vi "环动报警队列存储.vi"   [LabVIEW 2016, in "环境动力监测库.lvlib"]
types:
  T1 = cluster{"时间标识":timestamp, "设备":string, "日志信息":string}
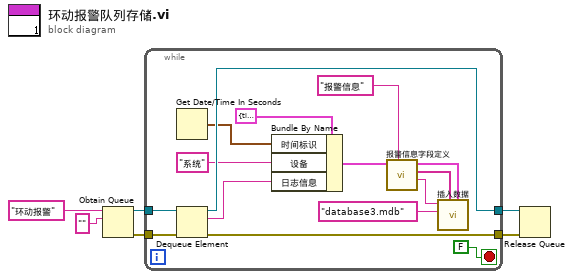
[diagram p0: block diagram]
diagram:
  n1 = Obtain Queue(name (unnamed)="环动报警" ("名称（未命名）"), element data type="" ("报警内容")) -> (queue out=w6:refnum<queue>, error out=w5:errorcluster)  [unwired: 3 in, 1 out]
  n2 = while {
    tunnel: w6 -> [w21]
    tunnel: w5 -> [w20]
    tunnel: [w18] -> w3
    tunnel: [w17] -> w2
    stop <- FALSE stop-if-true
    n3 = Get Date/Time In Seconds() -> (seconds since 1Jan1904=w9:timestamp)
    n4 = Dequeue Element(queue=w21, error in (no error)=w20) -> (queue out=w18:refnum<queue>, element=w7:string, error out=w17:errorcluster)  [unwired: 1 in, 1 out]
    n5 = Bundle By Name(cluster=T1 {"时间标识"=timestamp(0 s since 1904-01-01), "设备"="", "日志信息"=""} ("data in"), "时间标识"=w9, "设备"="系统", "日志信息"=w7) -> (w10:T1)
    n6 = call "报警信息字段定义.vi"("table输入"="报警信息", "data in"=w10) -> ("table输出"=w14:string, "columns"=w15:string[], "data out"=w16:T1)  [unwired: 7 in]
    n7 = call "插入数据.vi"("data"=w16, "columns"=w15, "database"="database3.mdb", "table"=w14) -> ()  [unwired: 7 in, 1 out]
  }
  n8 = Release Queue(queue=w3, error in (no error)=w2) -> ()  [unwired: 1 in, 3 out]
